vi "Ejercicio Sensores.vi"() -> ()   [LabVIEW 2020]
panel:
  out "Indicador T2":string
  out "Indicador T1":string
  out "Alarma T2":bool
  out "Alarma T1":bool
  in  "Umbral para T2":u8(slide) scale=0.0..100.0
  in  "Simular T2":dbl(knob) scale=0.0..100.0
  out "Termocupla 2 Tipo K":dbl(slide) scale=0.0..100.0
  in  "Umbral para T1":u8(slide) scale=0.0..100.0
  in  "Simular T1":dbl(knob) scale=0.0..100.0
  out "Termocupla 1 Tipo K":dbl(slide) scale=0.0..100.0
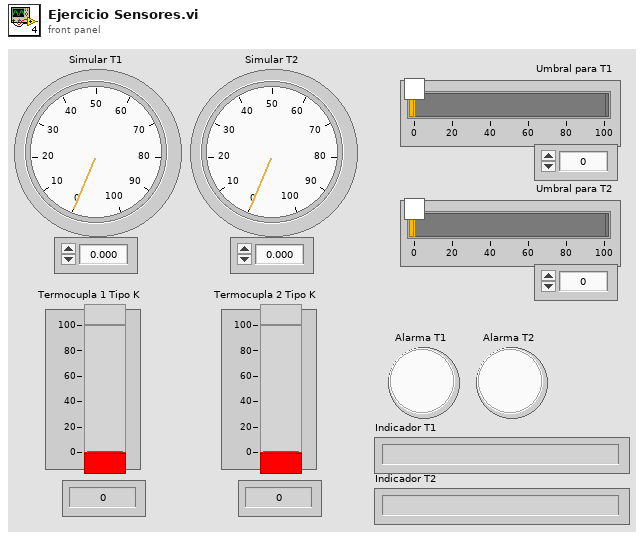
[diagram p1: front panel]
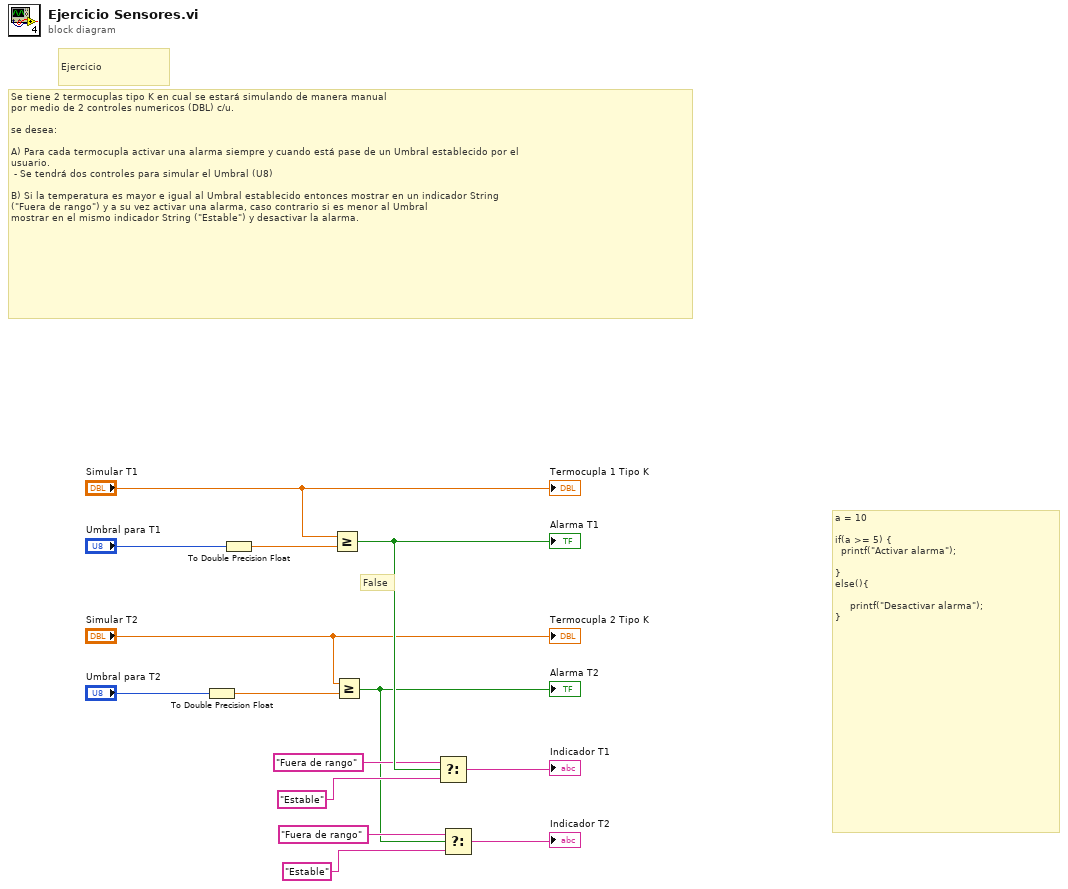
[diagram p0: block diagram]
diagram:
  # "False"
  # "a = 10\n\nif(a >= 5) {\n  printf(\"Activar alarma\");\n\n}\nelse(){\n\n     printf(\"Desactivar alarma\");\n}"
  # "Se tiene 2 termocuplas tipo K en cual se estará simulando de manera manual\npor medio de 2 controles numericos (DBL) c/u.\n\nse desea:\n\nA) Para cada termocupla activar una alarma siempre y cuando está pase de un Umbral establecido por el\nusuario.\n - Se tendrá dos controles para simular el Umbral (U8)\n\nB) Si la temperatura es mayor e igual al Umbral establecido entonces mostrar en un indicador String \n(\"Fuera de rango\") y a su vez activar una alarma, caso contrario si es menor al Umbral\nmostrar en el mismo indicador String (\"Estable\") y desactivar la alarma."
  # "Ejercicio"
  n1 = To Double Precision Float(number="Umbral para T2") -> (double precision float=w5:dbl)
  n2 = To Double Precision Float(number="Umbral para T1") -> (double precision float=w12:dbl)
  n3 = Greater Or Equal?(x="Simular T1", y=w12) -> (x >= y?=w11:bool)
  "Alarma T1" <- w11
  n4 = Greater Or Equal?(x="Simular T2", y=w5) -> (x >= y?=w2:bool)
  "Alarma T2" <- w2
  n5 = Select(t="Fuera de rango", s=w11, f="Estable") -> (s? t:f=→"Indicador T1":string)
  n6 = Select(t="Fuera de rango", s=w2, f="Estable") -> (s? t:f=→"Indicador T2":string)
  "Termocupla 1 Tipo K" <- "Simular T1"
  "Termocupla 2 Tipo K" <- "Simular T2"
